vi "Begin.vi"() -> (0 "error out":errorcluster)   [LabVIEW 2013]
doc: "Called before other user functions, this VI is expected to open initial I/O refnums, load in file data, and do all program initialization. Notice that the <B>error out</B> terminal is simply used for data flow. Wiring it to other structures or subVIs ensures that this VI runs first."
uses:
  <vilib>/Rock Robotics/SystemInterfaces/DIO/FPGA_DIOPWMChannel.ctl
  <vilib>/Rock Robotics/WPI/Joystick/WPI_JoystickDeviceEnum.ctl
  <vilib>/Rock Robotics/WPI/Camera/WPI_CameraImageSize.ctl
  <vilib>/Rock Robotics/SystemInterfaces/DIO/FPGA_DIOChannel.ctl
  <vilib>/Rock Robotics/WPI/Camera/WPI_CameraFrameRate.ctl
  <vilib>/Rock Robotics/WPI/RobotDrive/WPI_RobotDriveOpen2MotorWithVictor.vi
  <vilib>/Rock Robotics/WPI/MotorControl/WPI_MotorControlOpen Jaguar.vi
  <vilib>/Rock Robotics/WPI/MotorControl/WPI_MotorControlOpen Victor.vi
  <vilib>/Rock Robotics/WPI/Counter/WPI_CounterDigitalInputToDigitalSource.vi
  <vilib>/Rock Robotics/WPI/Counter/WPI_CounterOpen UpDown Mode.vi
panel:
  # "Shooter Encoder"
  # "Drive Encoder 2"
  # "Drive Encoder 1"
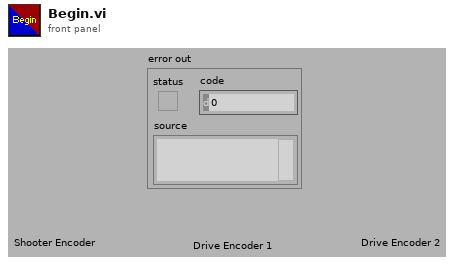
[diagram p1: front panel]
types:
  T1 = typedef "WPI_CameraFrameRate.ctl" = u32
  T2 = typedef "FPGA_DIOChannel.ctl" = enum8{"DIO 1", "DIO 2", "DIO 3", "DIO 4", "DIO 5", "DIO 6", "DIO 7", "DIO 8", "DIO 9", "DIO 10", "DIO 11", "DIO 12", "DIO 13", "DIO 14", "Invalid"}
  T3 = typedef "FPGA_DIOPWMChannel.ctl" = enum8{"PWM 1", "PWM 2", "PWM 3", "PWM 4", "PWM 5", "PWM 6", "PWM 7", "PWM 8", "PWM 9", "PWM 10", "Invalid"}
  T4 = typedef "WPI_JoystickDeviceEnum.ctl" = enum16{"USB 1", "USB 2", "USB 3", "USB 4", "Kinect 1", "Kinect 2"}
  T5 = typedef "WPI_CameraImageSize.ctl" = enum16{"640x480", "320x240", "160x120"}
  T6 = typedef "WPI_MotorControlDeviceRef.ctl" = cluster{"DeviceStatus":errorcluster, "Type":enum16{"PWM", "CAN"}, "PWM":cluster{"Digital Module":T7, "PWM Channel":T3, "DeadBand":T8}, "CAN":cluster{"Device Number":u8, "Control Mode":T9, "Semaphore":T10, "Max Vout":dbl}, "Invert":bool, "TransformRef":T11, "InvTransformRef":T11}
  T7 = typedef "FPGA_TypedefDigitalModule.ctl" = enum16{"Digital Module 1", "Digital Module 2"}
  T8 = typedef "WPI_PWMDeadband.ctl" = cluster{"Name":string, "maxPositivePwm":i32, "minPositivePwm":i32, "centerPwm":i32, "maxNegativePwm":i32, "minNegativePwm":i32, "angularRange":u16}
  T9 = typedef "WPI_CANJaguar_ControlMode.ctl" = enum8{"Percent VBus", "Current", "Speed", "Position", "Voltage"}
  T10 = typedef "Semaphore RefNum" = refnum<k1>
  T11 = typedef "WPI_PWMTransform_ConPane.ctl" = refnum<vi>
  T12 = typedef "WPI_JoystickDevRef.ctl" = cluster{"Device":T4}
  T13 = typedef "WPI_CameraDevRef.ctl" = cluster{"Camera Address":string, "CameraStatus":errorcluster, "Acquire Image Notifier":refnum<notifier>}
  T14 = typedef "WPI_DigitalInputDevRef.ctl" = cluster{"DevStatus":errorcluster, "DIO Channel":T2, "Digital Module":T7}
  T15 = typedef "FPGA_CounterEncoderSourceConvertionLVSourceType.ctl" = cluster{"DevStatus":errorcluster, "AnalogTriggerMode?":bool, "DigitalMode":cluster{"Digital Module":T7, "DIO Channel":T16}, "AnalogTriggerMode":cluster{"AnalogTriggerIndex":T17, "OutputType":T18}}
  T16 = typedef "FPGA_DIODigitalSourceChannel.ctl" = enum8{"DIO 1", "DIO 2", "DIO 3", "DIO 4", "DIO 5", "DIO 6", "DIO 7", "DIO 8", "DIO 9", "DIO 10", "DIO 11", "DIO 12", "DIO 13", "DIO 14", "Disabled"}
  T17 = typedef "FPGA_AnalogTriggerIndex.ctl" = enum8{"Trig 0", "Trig 1", "Trig 2", "Trig 3", "Trig 4", "Trig 5", "Trig 6", "Trig 7", "Invalid"}
  T18 = typedef "FPGA_AnalogTriggerOutType.ctl" = enum16{"InWindow", "TriggerState", "Rising", "Falling"}
  T19 = typedef "WPI_CounterDevRef.ctl" = cluster{"DevStatus":errorcluster, "CntIndex":T20}
  T20 = typedef "FPGA_CounterCtrSystemIndex.ctl" = enum8{"Ctr 0", "Ctr 1", "Ctr 2", "Ctr 3", "Ctr 4", "Ctr 5", "Ctr 6", "Ctr 7", "Invalid"}
  T21 = typedef "WPI_RobotDriveDevRef.ctl" = cluster{"DevStatus":errorcluster, "Motors[]":T6[], "Square Inputs":bool, "Max Output":dbl, "Isochronous":bool}
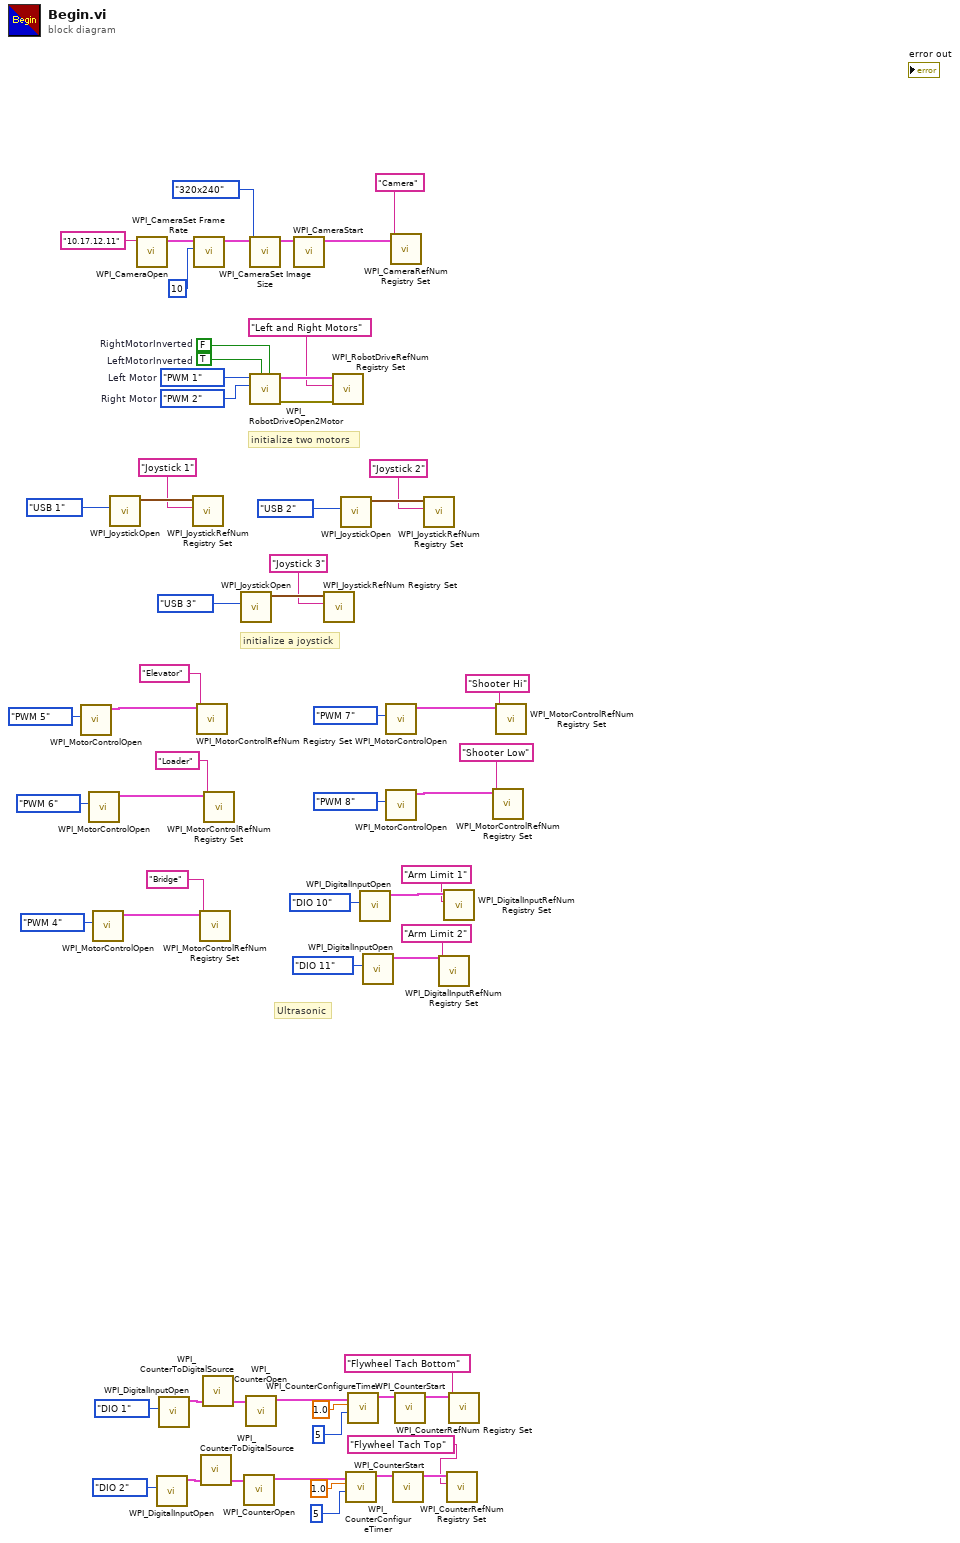
[diagram p0: block diagram]
diagram:
  w55 = FPGA_DIOPWMChannel."PWM 2"  # Right Motor
  w56 = FPGA_DIOPWMChannel."PWM 1"  # Left Motor
  w62 = TRUE  # LeftMotorInverted
  w63 = FALSE  # RightMotorInverted
  # "Ultrasonic"
  # "initialize a joystick"
  # "initialize two motors"
  n1 = call-poly <vilib>:"WPI_MotorControlOpen.vi"("PWM Channel"=FPGA_DIOPWMChannel."PWM 5") -> ("MotorControlDeviceRef"=w37:T6)  [unwired: 9 in, 1 out]
  n2 = call-poly <vilib>:"WPI_MotorControlOpen.vi"("PWM Channel"=FPGA_DIOPWMChannel."PWM 6") -> ("MotorControlDeviceRef"=w35:T6)  [unwired: 9 in, 1 out]
  n3 = call-poly <vilib>:"WPI_MotorControlOpen.vi"("PWM Channel"=FPGA_DIOPWMChannel."PWM 4") -> ("MotorControlDeviceRef"=w28:T6)  [unwired: 9 in, 1 out]
  n4 = call <vilib>:"WPI_JoystickOpen.vi"("JoystickDevice"=WPI_JoystickDeviceEnum."USB 1") -> ("JoystickDevRef"=w59:T12)  [unwired: 10 out]
  n5 = call <vilib>:"WPI_CameraOpen.vi"("Camera Address"="10.17.12.11") -> ("CameraDevRef"=w52:T13)  [unwired: 1 in, 9 out]
  n6 = call <vilib>:"WPI_DigitalInputOpen.vi"("DIO Channel"=FPGA_DIOChannel."DIO 2") -> ("DigitalInputDevRef"=w4:T14)  [unwired: 9 in, 1 out]
  n7 = call <vilib>:"WPI_DigitalInputOpen.vi"("DIO Channel"=FPGA_DIOChannel."DIO 1") -> ("DigitalInputDevRef"=w20:T14)  [unwired: 9 in, 1 out]
  n8 = call <vilib>:"WPI_JoystickRefNum Registry Set.vi"("refnum name"="Joystick 1", "JoystickDevRef"=w59) -> ()  [unwired: 1 in, 9 out]
  n9 = call <vilib>:"WPI_CameraSet Frame Rate.vi"("Frame Rate (fps)"=T1 10, "CameraDevRef"=w52) -> ("CameraDevRef Out"=w53:T13)  [unwired: 1 in, 8 out]
  n10 = call <vilib>:"WPI_MotorControlRefNum Registry Set.vi"("refnum name"="Elevator", "MotorControlDevRef"=w37) -> ()  [unwired: 8 in, 2 out]
  n11 = call <vilib>:"WPI_MotorControlRefNum Registry Set.vi"("refnum name"="Bridge", "MotorControlDevRef"=w28) -> ()  [unwired: 8 in, 2 out]
  n12 = call-poly <vilib>:"WPI_CounterToDigitalSource.vi"("DigitalInputDevRef"=w4) -> ("Digital Source"=w5:T15)  [unwired: 6 in]
  n13 = call-poly <vilib>:"WPI_CounterToDigitalSource.vi"("DigitalInputDevRef"=w20) -> ("Digital Source"=w19:T15)  [unwired: 6 in]
  n14 = call <vilib>:"WPI_MotorControlRefNum Registry Set.vi"("refnum name"="Loader", "MotorControlDevRef"=w35) -> ()  [unwired: 8 in, 2 out]
  n15 = call <vilib>:"WPI_JoystickOpen.vi"("JoystickDevice"=WPI_JoystickDeviceEnum."USB 3") -> ("JoystickDevRef"=w44:T12)  [unwired: 10 out]
  n16 = call-poly <vilib>:"WPI_CounterOpen.vi"("Up Source"=w5) -> ("CounterDevRef"=w7:T19)  [unwired: 9 in, 1 out]
  n17 = call-poly <vilib>:"WPI_CounterOpen.vi"("Up Source"=w19) -> ("CounterDevRef"=w17:T19)  [unwired: 9 in, 1 out]
  n18 = call <vilib>:"WPI_CameraSet Image Size.vi"("Image Size"=WPI_CameraImageSize."320x240", "CameraDevRef"=w53) -> ("CameraDevRef Out"=w51:T13)  [unwired: 1 in, 8 out]
  n19 = call-poly <vilib>:"WPI_RobotDriveOpen2Motor.vi"("Right Motor Inverted"=w63, "Left Motor Inverted"=w62, "Right Motor"=w55, "Left Motor"=w56) -> ("error out"=w57:errorcluster, "RobotDriveDevRef"=w61:T21)  [unwired: 1 in, 5 out]
  n20 = call <vilib>:"WPI_CameraStart.vi"("CameraDevRef"=w51) -> ("CameraDevRef Out"=w48:T13)  [unwired: 1 in, 9 out]
  n21 = call <vilib>:"WPI_JoystickRefNum Registry Set.vi"("refnum name"="Joystick 3", "JoystickDevRef"=w44) -> ()  [unwired: 1 in, 9 out]
  n22 = call <vilib>:"WPI_RobotDriveRefNum Registry Set.vi"("error in (no error)"=w57, "refnum name"="Left and Right Motors", "RobotDriveDevRef"=w61) -> ()  [unwired: 9 out]
  n23 = call <vilib>:"WPI_JoystickOpen.vi"("JoystickDevice"=WPI_JoystickDeviceEnum."USB 2") -> ("JoystickDevRef"=w47:T12)  [unwired: 10 out]
  n24 = call <vilib>:"WPI_CounterConfigureTimer.vi"("Number Samples to Average"=u8 5, "MaxPeriod (sec)"=1.0, "CounterDevRef in"=w7) -> ("CounterDevRef out"=w10:T19)  [unwired: 7 in, 1 out]
  n25 = call <vilib>:"WPI_CounterConfigureTimer.vi"("Number Samples to Average"=u8 5, "MaxPeriod (sec)"=1.0, "CounterDevRef in"=w17) -> ("CounterDevRef out"=w14:T19)  [unwired: 7 in, 1 out]
  n26 = call <vilib>:"WPI_DigitalInputOpen.vi"("DIO Channel"=FPGA_DIOChannel."DIO 10") -> ("DigitalInputDevRef"=w26:T14)  [unwired: 9 in, 1 out]
  n27 = call <vilib>:"WPI_DigitalInputOpen.vi"("DIO Channel"=FPGA_DIOChannel."DIO 11") -> ("DigitalInputDevRef"=w24:T14)  [unwired: 9 in, 1 out]
  n28 = call-poly <vilib>:"WPI_MotorControlOpen.vi"("PWM Channel"=FPGA_DIOPWMChannel."PWM 7") -> ("MotorControlDeviceRef"=w33:T6)  [unwired: 9 in, 1 out]
  n29 = call-poly <vilib>:"WPI_MotorControlOpen.vi"("PWM Channel"=FPGA_DIOPWMChannel."PWM 8") -> ("MotorControlDeviceRef"=w31:T6)  [unwired: 9 in, 1 out]
  n30 = call <vilib>:"WPI_CameraRefNum Registry Set.vi"("refnum name"="Camera", "CameraDevRef"=w48) -> ()  [unwired: 8 in, 2 out]
  n31 = call <vilib>:"WPI_CounterStart.vi"("CounterDevRef in"=w10) -> ("CounterDevRef out"=w11:T19)  [unwired: 9 in, 1 out]
  n32 = call <vilib>:"WPI_CounterStart.vi"("CounterDevRef in"=w14) -> ("CounterDevRef out"=w13:T19)  [unwired: 9 in, 1 out]
  n33 = call <vilib>:"WPI_JoystickRefNum Registry Set.vi"("refnum name"="Joystick 2", "JoystickDevRef"=w47) -> ()  [unwired: 1 in, 9 out]
  n34 = call <vilib>:"WPI_DigitalInputRefNum Registry Set.vi"("refnum name"="Arm Limit 2", "DigitalInputDevRef"=w24) -> ()  [unwired: 8 in, 2 out]
  n35 = call <vilib>:"WPI_DigitalInputRefNum Registry Set.vi"("refnum name"="Arm Limit 1", "DigitalInputDevRef"=w26) -> ()  [unwired: 8 in, 2 out]
  n36 = call <vilib>:"WPI_CounterRefNum Registry Set.vi"("refnum name"="Flywheel Tach Top", "CounterDevRef"=w11) -> ()  [unwired: 8 in, 2 out]
  n37 = call <vilib>:"WPI_CounterRefNum Registry Set.vi"("refnum name"="Flywheel Tach Bottom", "CounterDevRef"=w13) -> ()  [unwired: 8 in, 2 out]
  n38 = call <vilib>:"WPI_MotorControlRefNum Registry Set.vi"("refnum name"="Shooter Low", "MotorControlDevRef"=w31) -> ()  [unwired: 8 in, 2 out]
  n39 = call <vilib>:"WPI_MotorControlRefNum Registry Set.vi"("refnum name"="Shooter Hi", "MotorControlDevRef"=w33) -> ()  [unwired: 8 in, 2 out]
